vi "Clear Specific Error.vi"(8 "error in (no error)":errorcluster, 11 "error (0)":i32) -> (0 "error out":errorcluster)   [LabVIEW 2019, in "SEECD Engine.lvlib"]
doc: "Resets the error status to no error, code to 0, and source to an empty string if the error code matches \"error\"."
uses:
  SEECD Engine.lvlib
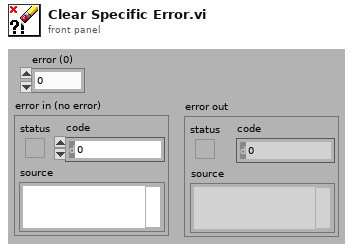
[diagram p1: front panel]
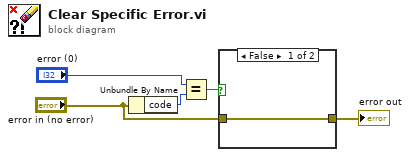
[diagram p0: block diagram]
diagram:
  n1 = Unbundle By Name("error in (no error)") -> ("code"=w3:i32)
  n2 = Equal?(x="error (0)", y=w3) -> (x = y?=w2:bool)
  n3 = case shown="False" w2 {
    tunnel: "error in (no error)" -> [w6 _]
    tunnel: [w6 _] -> w4
    frame False {
    }
    frame True {
    }
  }
  "error out" <- w4
